vi "Recursive Parse XML Priv.vi"(5 "Data Types Dict":variant, 7 "Parent ID (empty)":string, 8 "Error In":errorcluster, 10 "XML String":string, 11 "Tree Dict":variant) -> (0 "Error Out":errorcluster, 2 "XML String":string, 3 "Tree Dict Out":variant)   [LabVIEW 2017, in "Tree API.lvlib" / "Tree.lvclass"]
uses:
  Tree.lvclass
  <vilib>/ErrorRing/Error Ring.xnode
  <vilib>/Utility/error.llb/Error Cluster From Error Code.vi
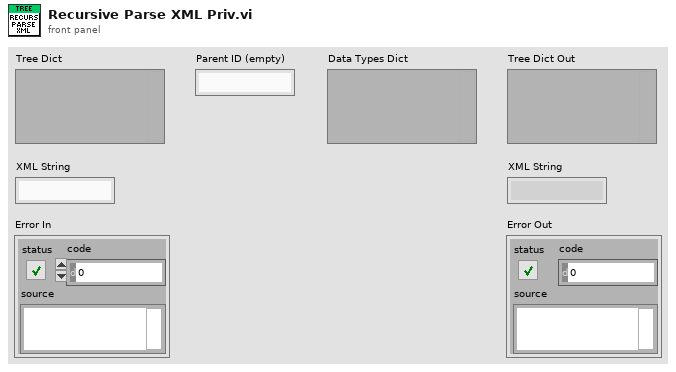
[diagram p1: front panel]
types:
  T1 = typedef "Tree API.lvlib/Tree.lvclass/Parsing Info.ctl" = cluster{"</ Tag>":bool, "<Tag />":bool, "Nothing Found":bool, "Ignore":bool}
  T2 = typedef "Tree API.lvlib/Tree.lvclass/Parsed Header.ctl" = cluster{"Tag Name":string, "Attr Names":string[], "Attr Vals":string[], "Has Type":bool}
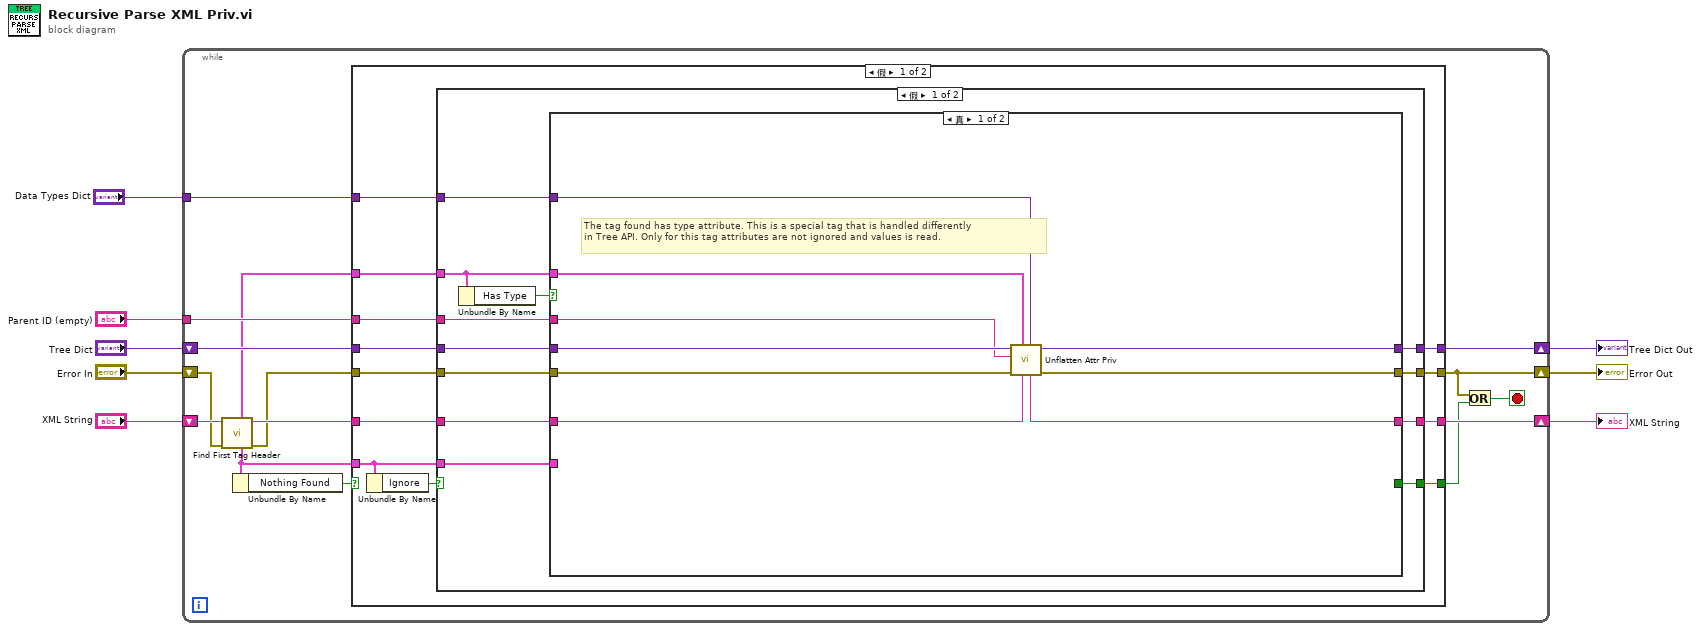
[diagram p0: block diagram]
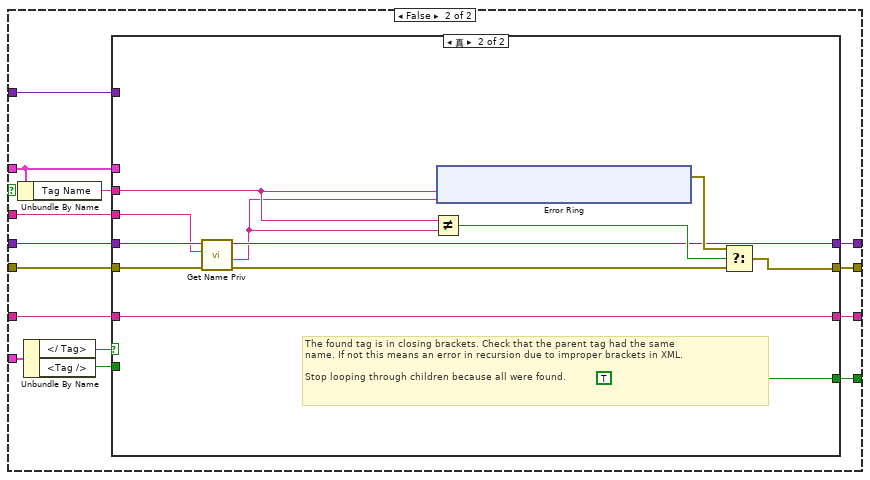
[diagram p2: hidden frame]
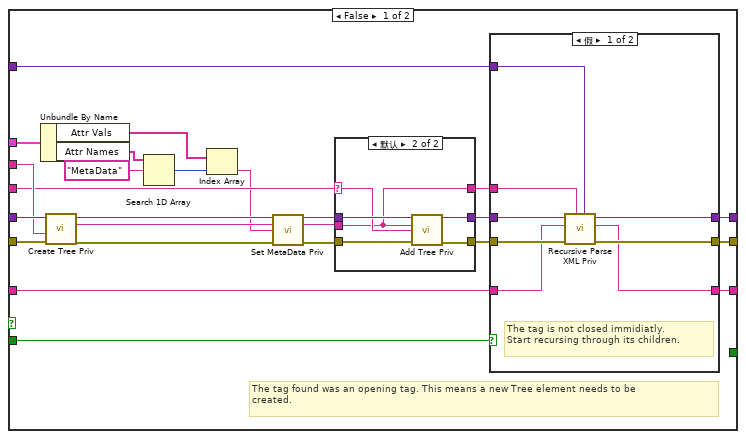
[diagram p3: hidden frame]
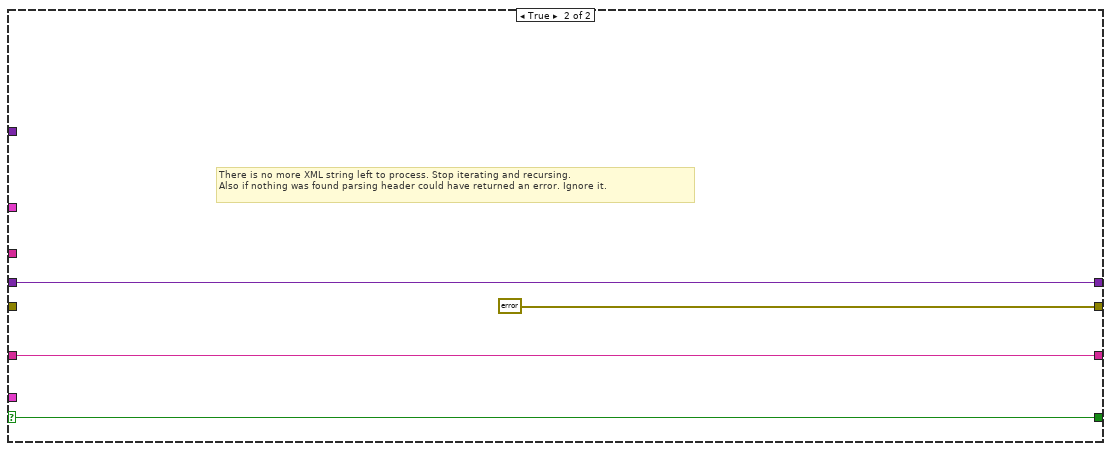
[diagram p7: hidden frame]
diagram:
  n1 = while {
    tunnel: "Parent ID (empty)" -> [w23]
    shift-right: [w21] -> w3
    shift-left: "Tree Dict" -> [w22]
    shift-right: [w18] -> w7
    shift-left: "Error In" -> [w11]
    shift-right: [w19] -> w5
    shift-left: "XML String" -> [w20]
    tunnel: "Data Types Dict" -> [w9]
    stop <- w16 stop-if-true
    n2 = call "Find First Tag Header.vi"("Error In"=w11, "XML String"=w20) -> ("Error Out"=w10:errorcluster, "After First Tag String"=w13:string, "Parsing Info"=w15:T1, "Parsed Header"=w12:T2)  [unwired: 6 in]
    n3 = Unbundle By Name(w15) -> ("Nothing Found"=w14:bool)
    n4 = case shown="假" w14 {
      selector: w14 -> [_ w139]
      tunnel: w23 -> [w35 _]
      tunnel: w22 -> [w34 w141]
      tunnel: [w33 errorcluster {"status"=FALSE, "code"=0, "source"=""} ("Error Out")] -> w18
      tunnel: [w32 w141] -> w21
      tunnel: w10 -> [w31 _]
      tunnel: w15 -> [w26 _]
      tunnel: [w29 w139] -> w17
      tunnel: [w30 w140] -> w19
      tunnel: w13 -> [w28 w140]
      tunnel: w12 -> [w27 _]
      tunnel: w9 -> [w24 _]
      frame False {
        n5 = Unbundle By Name(w26) -> ("Ignore"=w25:bool)
        n6 = case shown="假" w25 {
          tunnel: w35 -> [w47 _]
          tunnel: w34 -> [w46 w136]
          tunnel: [w45 w135] -> w33
          tunnel: [w44 w136] -> w32
          tunnel: w31 -> [w43 w135]
          tunnel: [w42 w137] -> w30
          tunnel: [w41 _] -> w29
          tunnel: w28 -> [w40 w137]
          tunnel: w27 -> [w37 _]
          tunnel: w26 -> [w39 _]
          tunnel: w24 -> [w36 _]
          frame False {
            n7 = Unbundle By Name(w37) -> ("Has Type"=w38:bool)
            n8 = case shown="真" w38 {
              tunnel: w47 -> [w48 w70]
              tunnel: w46 -> [w52 w69]
              tunnel: [w54 w63] -> w45
              tunnel: [w55 w64] -> w44
              tunnel: w43 -> [w53 w68]
              tunnel: w39 -> [_ w67]
              tunnel: [w50 w62] -> w42
              tunnel: [_ w61] -> w41
              tunnel: w40 -> [w56 w60]
              tunnel: w37 -> [w49 w58]
              tunnel: w36 -> [w51 w59]
              frame True {
                # "The tag found has type attribute. This is a special tag that is handled differently\nin Tree API. Only for this tag attributes are not ignored and values is read."
                n9 = call "Unflatten Attr Priv.vi"("Data Types Dict"=w51, "After First Tag String"=w56, "Parsed Header"=w49, "error in"=w53, "Parent ID (empty)"=w48, "Tree Dict"=w52) -> ("error out"=w54:errorcluster, "Tree Dictionary Out"=w55:variant, "After First Tag String"=w50:string)  [unwired: 3 in]
              }
              frame False {
                n10 = Unbundle By Name(w58) -> ("Tag Name"=w57:string)
                n11 = Unbundle By Name(w67) -> ("</ Tag>"=w66:bool, "<Tag />"=w65:bool)
                n12 = case shown="真" w66 {
                  tunnel: w70 -> [w86 w118]
                  tunnel: w69 -> [w89 w120]
                  tunnel: w68 -> [w88 w119]
                  tunnel: w65 -> [w94 _]
                  tunnel: w57 -> [w87 w121]
                  tunnel: w60 -> [w93 w122]
                  tunnel: [w92 w117] -> w64
                  tunnel: [w91 w123] -> w63
                  tunnel: [w90 w122] -> w62
                  tunnel: [_ TRUE] -> w61
                  tunnel: w59 -> [w82 _]
                  tunnel: w58 -> [w81 _]
                  frame False {
                    # "The tag found was an opening tag. This means a new Tree element needs to be\ncreated."
                    n13 = Unbundle By Name(w81) -> ("Attr Vals"=w77:string[], "Attr Names"=w78:string[])
                    n14 = call "Create Tree Priv.vi"("Error In"=w88, "Name"=w87, "Tree Dictionary In"=w89) -> ("Error Out"=w71:errorcluster, "Unique ID"=w73:string, "Tree Dictionary Out"=w76:variant)  [unwired: 6 in]
                    n15 = Search 1D Array(1D array=w78, element="MetaData") -> (index of element=w80:i32)  [unwired: 1 in]
                    n16 = Index Array(array=w77, index=w80) -> (element=w72:string)
                    n17 = call "Set MetaData Priv.vi"("Tree Dict"=w76, "Tree ID"=w73, "MetaData"=w72, "error in"=w71) -> ("Tree Dict"=w75:variant, "error out"=w74:errorcluster)  [unwired: 10 in]
                    n18 = case shown="默认" w86 {
                      selector: w86 -> [_ w102]
                      tunnel: w75 -> [w97 w103]
                      tunnel: w73 -> [w95 w98]
                      tunnel: w74 -> [w96 w101]
                      tunnel: [w97 w100] -> w85
                      tunnel: [w96 w99] -> w84
                      tunnel: [w95 w98] -> w83
                      frame "" {
                      }
                      frame Default {
                        n19 = call "Add Tree Priv.vi"("Tree Dictionary In"=w103, "Unique ID"=w98, "Parent ID"=w102, "Error In"=w101) -> ("Tree Dictionary Out"=w100:variant, "Error Out"=w99:errorcluster)  [unwired: 10 in]
                      }
                    }
                    n20 = case shown="假" w94 {
                      tunnel: w85 -> [w111 w114]
                      tunnel: w84 -> [w110 w113]
                      tunnel: w93 -> [w109 w112]
                      tunnel: [w108 w114] -> w92
                      tunnel: [w107 w113] -> w91
                      tunnel: w83 -> [w106 _]
                      tunnel: [w105 w112] -> w90
                      tunnel: w82 -> [w104 _]
                      frame False {
                        # "The tag is not closed immidiatly.\nStart recursing through its children."
                        n21 = call "Recursive Parse XML Priv.vi"("Data Types Dict"=w104, "Parent ID (empty)"=w106, "Error In"=w110, "XML String"=w109, "Tree Dict"=w111) -> ("Error Out"=w107:errorcluster, "XML String"=w105:string, "Tree Dict Out"=w108:variant)  [unwired: 4 in]
                      }
                      frame True {
                      }
                    }
                  }
                  frame True {
                    # "The found tag is in closing brackets. Check that the parent tag had the same\nname. If not this means an error in recursion due to improper brackets in XML.\n\nStop looping through children because all were found."
                    n22 = call "Get Name Priv.vi"("error in"=w119, "Unique ID"=w118, "Tree Dictionary"=w120) -> ("error out"=w115:errorcluster, "Name"=w116:string, "Tree Dictionary Out"=w117:variant)  [unwired: 6 in]
                    n23 = Not Equal?(x=w121, y=w116) -> (x != y?=w125:bool)
                    n24 = xnode "Error Ring"("参数 0"=w121, "参数 1"=w116) -> ("错误输出"=w124:errorcluster)
                    n25 = Select(t=w124, s=w125, f=w115) -> (s? t:f=w123:errorcluster)
                  }
                }
              }
            }
          }
          frame True {
          }
        }
      }
      frame True {
        # "There is no more XML string left to process. Stop iterating and recursing.\nAlso if nothing was found parsing header could have returned an error. Ignore it."
      }
    }
    n26 = Or(x=w18, y=w17) -> (x .or. y?=w16:bool)
  }
  "Error Out" <- w7
  "XML String" <- w5
  "Tree Dict Out" <- w3
